vi "global variable-一色累積次數.vi"() -> ()   [LabVIEW 2014]
panel:
  out "一色累積次數":i32
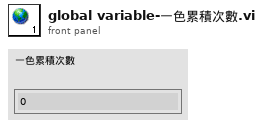
[diagram p1: front panel]
diagram:
